vi "Random Strip Chart.vi"() -> ()   [LabVIEW 2025]
panel:
  in  "Loop time (ms)":dbl(knob) scale=0.0..1000.0
  out "Waveform Chart":dbl(graph)
  in  "Stop":bool
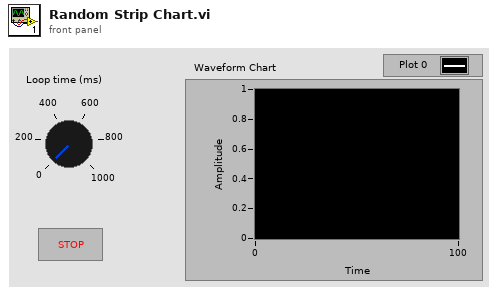
[diagram p1: front panel]
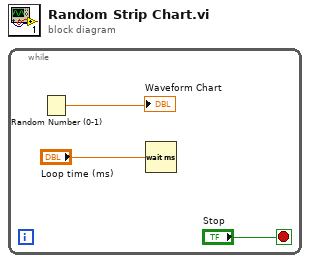
[diagram p0: block diagram]
diagram:
  n1 = while {
    stop <- "Stop" stop-if-true
    n2 = Random Number (0-1)() -> (number: 0 to 1=→"Waveform Chart":dbl)
    n3 = Wait (ms)(milliseconds to wait="Loop time (ms)") -> ()  [unwired: 1 out]
  }
